vi "motor_move_rotate.vi"(7 "旋转修正":dbl=1.0, 8 "错误输入（无错误）":errorcluster, 10 "目标转数":dbl, 11 "device index":T1) -> (0 "错误输出":errorcluster, 3 "当前转数":dbl)   [LabVIEW 2017]
doc: "本VI用于旋转磁铁，乘了一些系数做传动齿轮的修正,其中6与11是两个联动的齿轮直径比例，0.974 是实验上校准的传动误差。360是度数和圈数的一些单位转换。\n20170501\n修正了一下传动误差，0.977可能更加精确一些。"
uses:
  device index.ctl
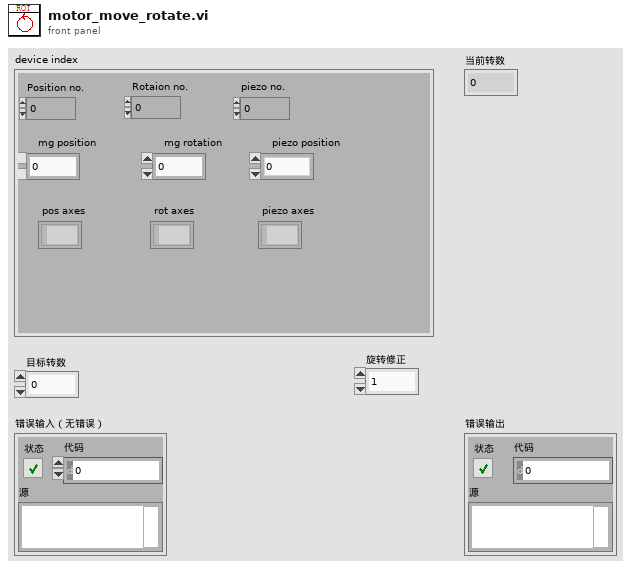
[diagram p1: front panel]
types:
  T1 = typedef "device index.ctl" = cluster{"Position no.":i32, "Rotaion no.":i32, "piezo no.":i32, "mg position":dbl, "mg rotation":dbl, "piezo position":dbl, "pos axes":string[], "rot axes":string[], "piezo axes":string[]}
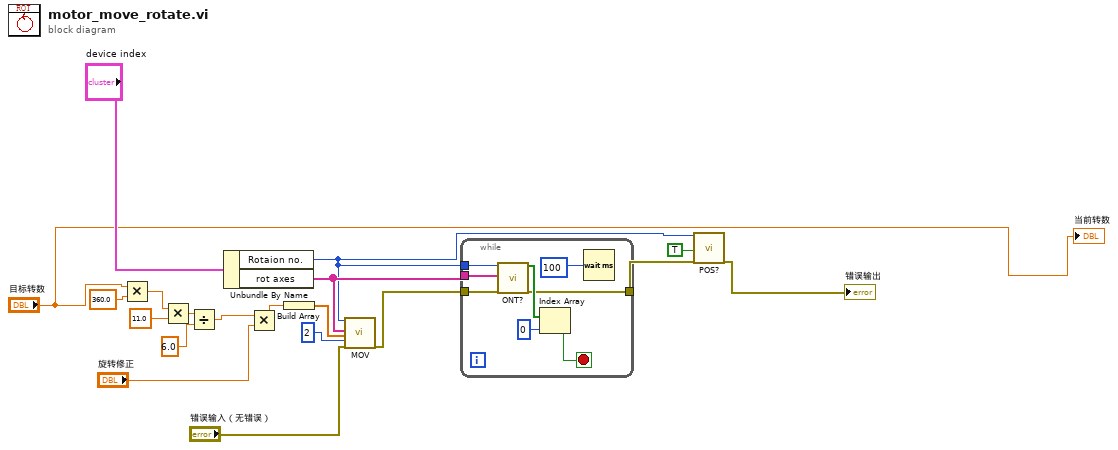
[diagram p0: block diagram]
diagram:
  n1 = Multiply(x="目标转数", y=360.0) -> (x*y=w8:dbl)
  n2 = Multiply(x=w8, y=11.0) -> (x*y=w6:dbl)
  n3 = Divide(x=w6, y=6.0) -> (x/y=w4:dbl)
  n4 = Unbundle By Name("device index") -> ("Rotaion no."=w15:i32, "rot axes"=w18:string[])
  n5 = Multiply(x=w4, y="旋转修正") -> (x*y=w3:dbl)
  n6 = Build Array(w3) -> (w9:dbl[])
  n7 = call "MOV.vi"("System no."=w15, "Axes to move"=w18, "Position values"=w9, "No.of digits"=i16 2, "error in"="错误输入（无错误）") -> ("error out"=w16:errorcluster)  [unwired: 14 in]
  n8 = while {
    tunnel: w15 -> [w27]
    tunnel: [w23] -> w17
    tunnel: w16 -> [w21]
    tunnel: w18 -> [w20]
    stop <- w24 stop-if-true
    n9 = call "ONT?.vi"("System no."=w27, "Axes to query"=w20, "error in"=w21) -> ("Axis on target?"=w26:bool[], "error out"=w23:errorcluster)  [unwired: 15 in]
    n10 = Index Array(array=w26, index=0 ("索引")) -> (element=w24:bool)
    n11 = Wait (ms)(milliseconds to wait=u32 100 ("等待时间（毫秒）")) -> ()  [unwired: 1 out]
  }
  n12 = call "POS?.vi"("System no."=w15, "All axes?"=TRUE, "error in"=w17) -> ("error out"=→"错误输出":errorcluster)  [unwired: 15 in, 1 out]
  "当前转数" <- "目标转数"
